vi "SENS_SEGM_BWID_RES_CONT_ON_OFF.vi"(0 "VISA IN":refnum<visa-resource-name>, 1 "BW Control ON/OFF":bool, 5 "error in":errorcluster, 7 "Channel":i32) -> (14 "VISA Out":refnum<visa-resource-name>, 19 "error out":errorcluster)   [LabVIEW 2018, in "PNA-X.lvlib"]
doc: "SENSe<cnum>:SEGMent:BWIDth[:RESolution]:CONTrol <ON | OFF> \n1806\n\n(Read-Write) Specifies whether the IF Bandwidth resolution can be set independently for each \nsegment. \nParameters \n<cnum> Any existing channel number. If unspecified, value is set to 1 \n<ON | OFF> ON (or 1) - turns Bandwidth control ON. Bandwidth can be set for each \nsegment \nOFF (or 0) - turns Bandwidth control OFF. Use channel bandwidth setting \nExamples SENS:SEGM:BWID:CONT ON \nsense2:segment:bwidth:control off \nQuery Syntax SENSe<cnum>:SEGMent:BWIDth[:RESolution]:CONTrol? \nReturn Type Boolean (1 = ON, 0 = OFF) \nDefault OFF"
uses:
  PNA-X.lvlib
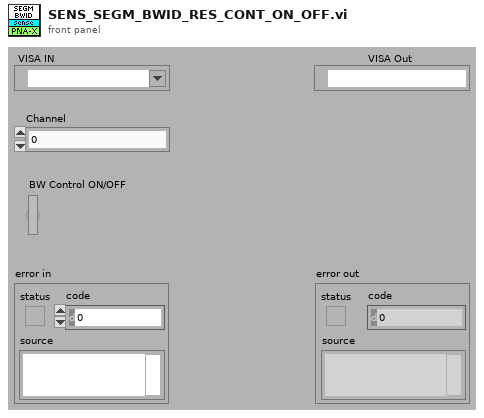
[diagram p1: front panel]
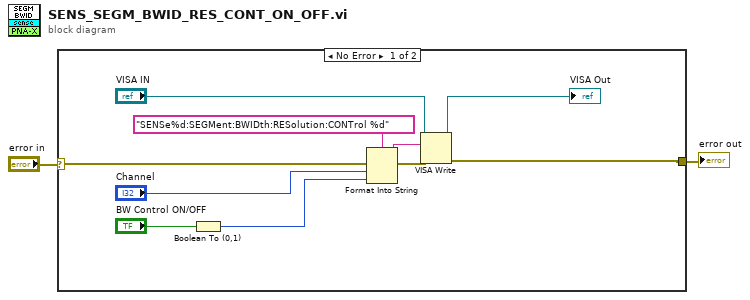
[diagram p0: block diagram]
diagram:
  n1 = case shown="No Error" "error in" {
    selector: "error in" -> [w12 w13]
    tunnel: [w7 w13] -> w1
    frame No Error {
      n2 = Boolean To (0,1)(Boolean="BW Control ON/OFF") -> (0, 1=w3:i16)
      n3 = Format Into String(format string="SENSe%d:SEGMent:BWIDth:RESolution:CONTrol %d" ("Cmdline"), error in=w12, "Channel", w3) -> (resulting string=w10:string, error out=w11:errorcluster)  [unwired: 1 in]
      n4 = VISA Write(VISA resource name="VISA IN", write buffer=w10, error in (no error)=w11) -> (VISA resource name out=→"VISA Out":refnum<visa-resource-name>, error out=w7:errorcluster)  [unwired: 1 out]
    }
    frame Error {
    }
  }
  "error out" <- w1
